vi "Update Path.vi"(8 "From":cluster{"Row":i32, "Col":i32}, 9 "gScore":i32, 10 "Position":cluster{"Row":i32, "Col":i32}, 11 "Map In":T1) -> (3 "Map":T1)   [LabVIEW 2022 SP3, in "AoC22.lvlib"]
uses:
  AoC22.lvlib
  Map.ctl
  <vilib>/Utility/miscctls.llb/LVMapReplaceAction.ctl
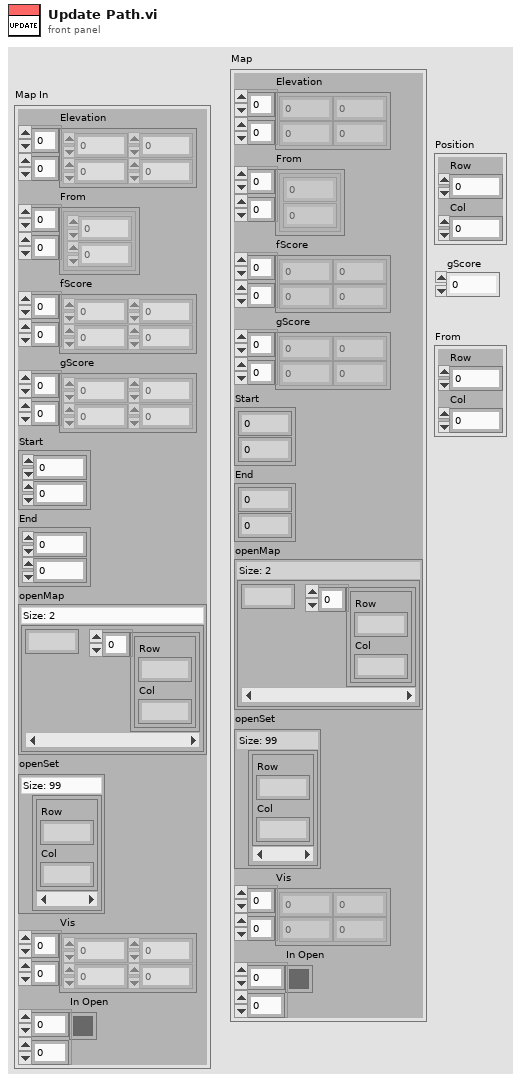
[diagram p1: front panel]
types:
  T1 = typedef "AoC22.lvlib/Map.ctl" = cluster{"Elevation":u8[][], "From":cluster{"Row":i32, "Col":i32}[][], "fScore":i32[][], "gScore":i32[][], "Start":cluster{"Row":i32, "Col":i32}, "End":cluster{"Row":i32, "Col":i32}, "openMap":map{i32, cluster{"Row":i32, "Col":i32}[]}, "openSet":set{cluster{"Row":i32, "Col":i32}}, "Vis":u8[][], "In Open":bool[][]}
  T2 = typedef "LVMapReplaceAction.ctl" = enum32{"Modify Entry only if found", "Add or Modify Entry", "Delete Entry"}
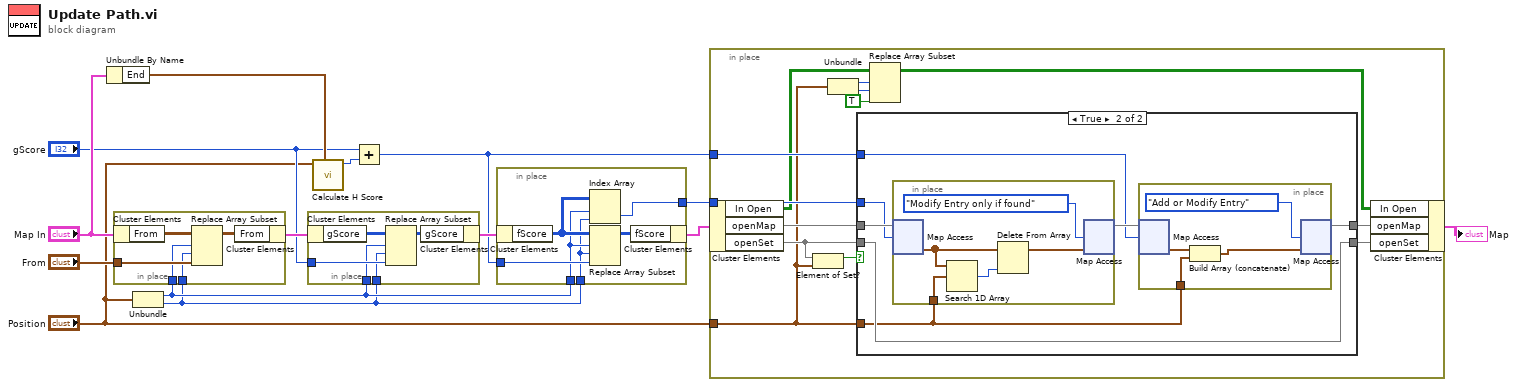
[diagram p0: block diagram]
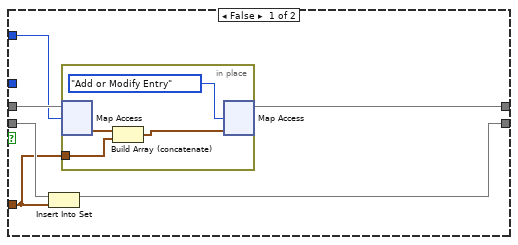
[diagram p2: hidden frame]
diagram:
  n1 = Unbundle By Name("Map In") -> ("End"=w11:cluster{"Row":i32, "Col":i32})
  n2 = Unbundle("Position") -> ("Row"=w7:i32, "Col"=w6:i32)
  n3 = in-place {
    in-place-border: "From" -> [w18]
    in-place-border: w7 -> [w17]
    in-place-border: w6 -> [w16]
    n4 = in-place-cluster #1("Map In") -> ("From"=w19:cluster{"Row":i32, "Col":i32}[][])
    n5 = Replace Array Subset(array=w19, new element=w18, index (row)=w17, index (col)=w16) -> (w15:cluster{"Row":i32, "Col":i32}[][])
    n6 = in-place-cluster #1("From"=w15) -> (w13:T1)
  }
  n7 = in-place {
    in-place-border: "gScore" -> [w23]
    in-place-border: w7 -> [w22]
    in-place-border: w6 -> [w21]
    n8 = in-place-cluster #2(w13) -> ("gScore"=w24:i32[][])
    n9 = Replace Array Subset(array=w24, new element=w23, index (row)=w22, index (col)=w21) -> (w20:i32[][])
    n10 = in-place-cluster #2("gScore"=w20) -> (w8:T1)
  }
  n11 = call "Calculate H Score.vi"("End"=w11, "Position"="Position") -> ("hScore"=w9:i32)  [unwired: 9 in]
  n12 = Add(x="gScore", y=w9) -> (x+y=w3:i32)
  n13 = in-place {
    in-place-border: w3 -> [w30]
    in-place-border: w7 -> [w27]
    in-place-border: w6 -> [w26]
    in-place-border: [w25] -> w2
    n14 = in-place-cluster #3(w8) -> ("fScore"=w28:i32[][])
    n15 = Index Array(array=w28, index (row)=w27, index (col)=w26) -> (element=w25:i32)
    n16 = Replace Array Subset(array=w28, new element=w30, index (row)=w27, index (col)=w26) -> (w29:i32[][])
    n17 = in-place-cluster #3("fScore"=w29) -> (w5:T1)
  }
  n18 = in-place {
    in-place-border: "Position" -> [w36]
    in-place-border: w3 -> [w40]
    in-place-border: w2 -> [w37]
    n19 = in-place-cluster #4(w5) -> ("In Open"=w34:bool[][], "openMap"=w41:map{i32, cluster{"Row":i32, "Col":i32}[]}, "openSet"=w42:set{cluster{"Row":i32, "Col":i32}})
    n20 = Element of Set?(10:w36, 11:w42) -> (3:w43:bool)
    n21 = Unbundle(w36) -> ("Row"=w35:i32, "Col"=w33:i32)
    n22 = case shown="True" w43 {
      tunnel: w42 -> [w49 w60]
      tunnel: w41 -> [w47 w59]
      tunnel: w36 -> [w45 w56]
      tunnel: w40 -> [w46 w55]
      tunnel: [w48 w60] -> w39
      tunnel: [w44 w54] -> w38
      tunnel: w37 -> [_ w58]
      frame False {
        n23 = Insert Into Set(10:w45, 11:w49) -> (3:w48:set{cluster{"Row":i32, "Col":i32}})  [unwired: 1 out]
        n24 = in-place {
          in-place-border: w45 -> [w52]
          n25 = in-place-map #5(w47, w46) -> (w53:cluster{"Row":i32, "Col":i32}[])  [unwired: 1 in, 1 out]
          n26 = Build Array (concatenate)(w53, w52) -> (w51:cluster{"Row":i32, "Col":i32}[])
          n27 = in-place-map #5(w51, LVMapReplaceAction."Add or Modify Entry" ("action")) -> (w44:map{i32, cluster{"Row":i32, "Col":i32}[]})  [unwired: 2 out]
        }
      }
      frame True {
        n28 = in-place {
          in-place-border: w56 -> [w69]
          n29 = in-place-map #6(w59, w58) -> (w68:cluster{"Row":i32, "Col":i32}[])  [unwired: 1 in, 1 out]
          n30 = Search 1D Array(1D array=w68, element=w69) -> (index of element=w67:i32)  [unwired: 1 in]
          n31 = Delete From Array(array=w68, index=w67) -> (array with subset deleted=w66:cluster{"Row":i32, "Col":i32}[])  [unwired: 1 in, 1 out]
          n32 = in-place-map #6(w66, LVMapReplaceAction."Modify Entry only if found" ("action")) -> (w57:map{i32, cluster{"Row":i32, "Col":i32}[]})  [unwired: 2 out]
        }
        n33 = in-place {
          in-place-border: w56 -> [w63]
          n34 = in-place-map #7(w57, w55) -> (w64:cluster{"Row":i32, "Col":i32}[])  [unwired: 1 in, 1 out]
          n35 = Build Array (concatenate)(w64, w63) -> (w62:cluster{"Row":i32, "Col":i32}[])
          n36 = in-place-map #7(w62, LVMapReplaceAction."Add or Modify Entry" ("action")) -> (w54:map{i32, cluster{"Row":i32, "Col":i32}[]})  [unwired: 2 out]
        }
      }
    }
    n37 = Replace Array Subset(array=w34, new element=TRUE ("new element/subarray"), index (row)=w35, index (col)=w33) -> (w31:bool[][])
    n38 = in-place-cluster #4("In Open"=w31, "openMap"=w38, "openSet"=w39) -> (→"Map":T1)
  }
